vi "SiPM_Characterization.vi"() -> ()   [LabVIEW 2015]
panel:
  in  "Nb of Pixels":u16
  in  "Stop":bool
  in  "Board_ID":string="1"
  in  "Scope Tests":bool
  in  "IV_Tests":bool
  in  "SiPM Model":string="s130"
  in  "SiPM Supplier":string="Hamamatsu_"
  in  "Save Reults to file":bool
  in  "Specify folder to save results":path=path "C:/Users/user/Dropbox/European_Space_Agency/Program_files/SiPM_Characterization/Data"
  # "NCSR\nDetectors\nInstrumentation\nLaboratory"
  # "Si PhotoMultiplier Characterization Tests"
  # "Device Under Test"
  # "Test Board"
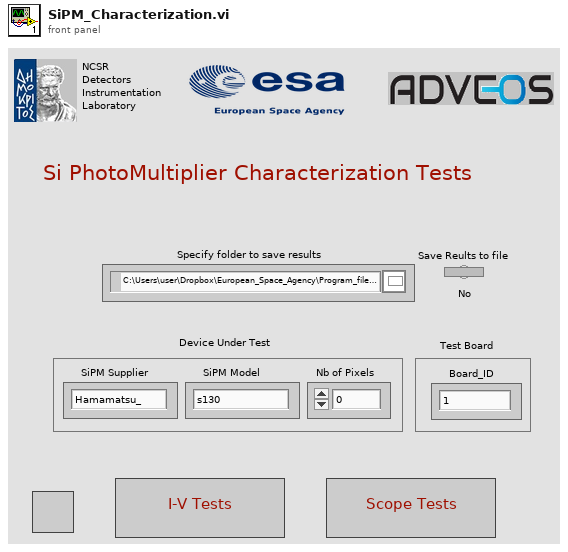
[diagram p1: front panel]
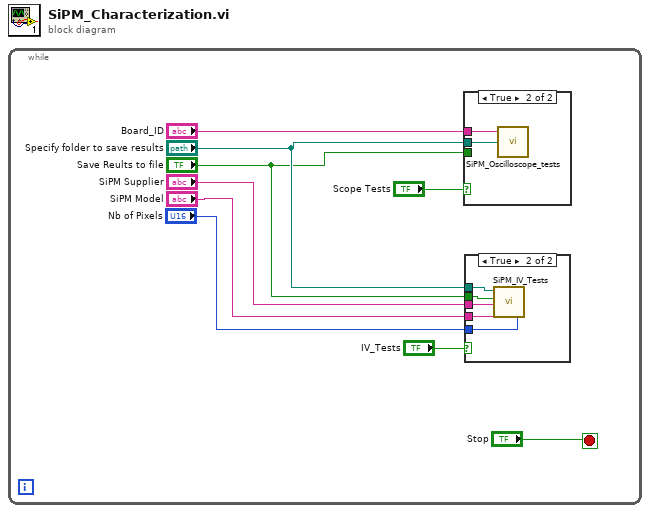
[diagram p0: block diagram]
diagram:
  n1 = while {
    stop <- "Stop" stop-if-true
    n2 = case shown="True" "Scope Tests" {
      tunnel: "Board_ID" -> [_ w16]
      tunnel: "Specify folder to save results" -> [_ w15]
      tunnel: "Save Reults to file" -> [_ _]
      frame False {
      }
      frame True {
        n3 = call "SiPM_Oscilloscope_tests.vi"("Results Directory"=w15, "Isotope"=w16) -> ()  [unwired: 1 in]
      }
    }
    n4 = case shown="True" "IV_Tests" {
      tunnel: "Specify folder to save results" -> [_ w14]
      tunnel: "Save Reults to file" -> [_ w13]
      tunnel: "SiPM Supplier" -> [_ w12]
      tunnel: "SiPM Model" -> [_ w11]
      tunnel: "Nb of Pixels" -> [_ w10]
      frame False {
      }
      frame True {
        n5 = call "SiPM_IV_Tests.vi"("Nb of Pixels"=w10, "SiPM Model"=w11, "SiPM Supplier"=w12, "Save Reults to file"=w13, "Specify folder to save results"=w14) -> ()  [unwired: 1 in]
      }
    }
  }
